vi "Find-NoClasses.vi"() -> ()   [LabVIEW 2016]
uses:
  D:/Users/blume/Desktop/LV/MongoDB-Driver/MLV DLLs/MongoLabVIEW.dll
  LV/MongoDB-Driver/MLV DLLs/MongoLabVIEW.dll
  HITRAN-Line-Cluster.ctl
panel:
  out "Lines":T1[](array[typedef]) {"trans_nu" format="%#.6g"}
  out "Find":string[](array[string])
  out "# lines":i32
  out "convertionTime (ms)":u32
  out "selectionTime (ms)":u32
  in  "selectionString":string="{ _id: false }"
  in  "filterString":string="{ trans_nu: { $gte: 7246, $lte: 7352 }, trans_molec_id: 1 }"
  in  "sortString":string="{param_intensity_weighted_abundace: -1}"
  in  "limitInteger":i32=100
  out "GetNumberOfDocs":i64
  in  "collectionName":string="hitran_2012"
  in  "databaseName":string="hitran"
  in  "connectionString":string="mongodb://tulpe:27017"
  # "MongoDB Example"
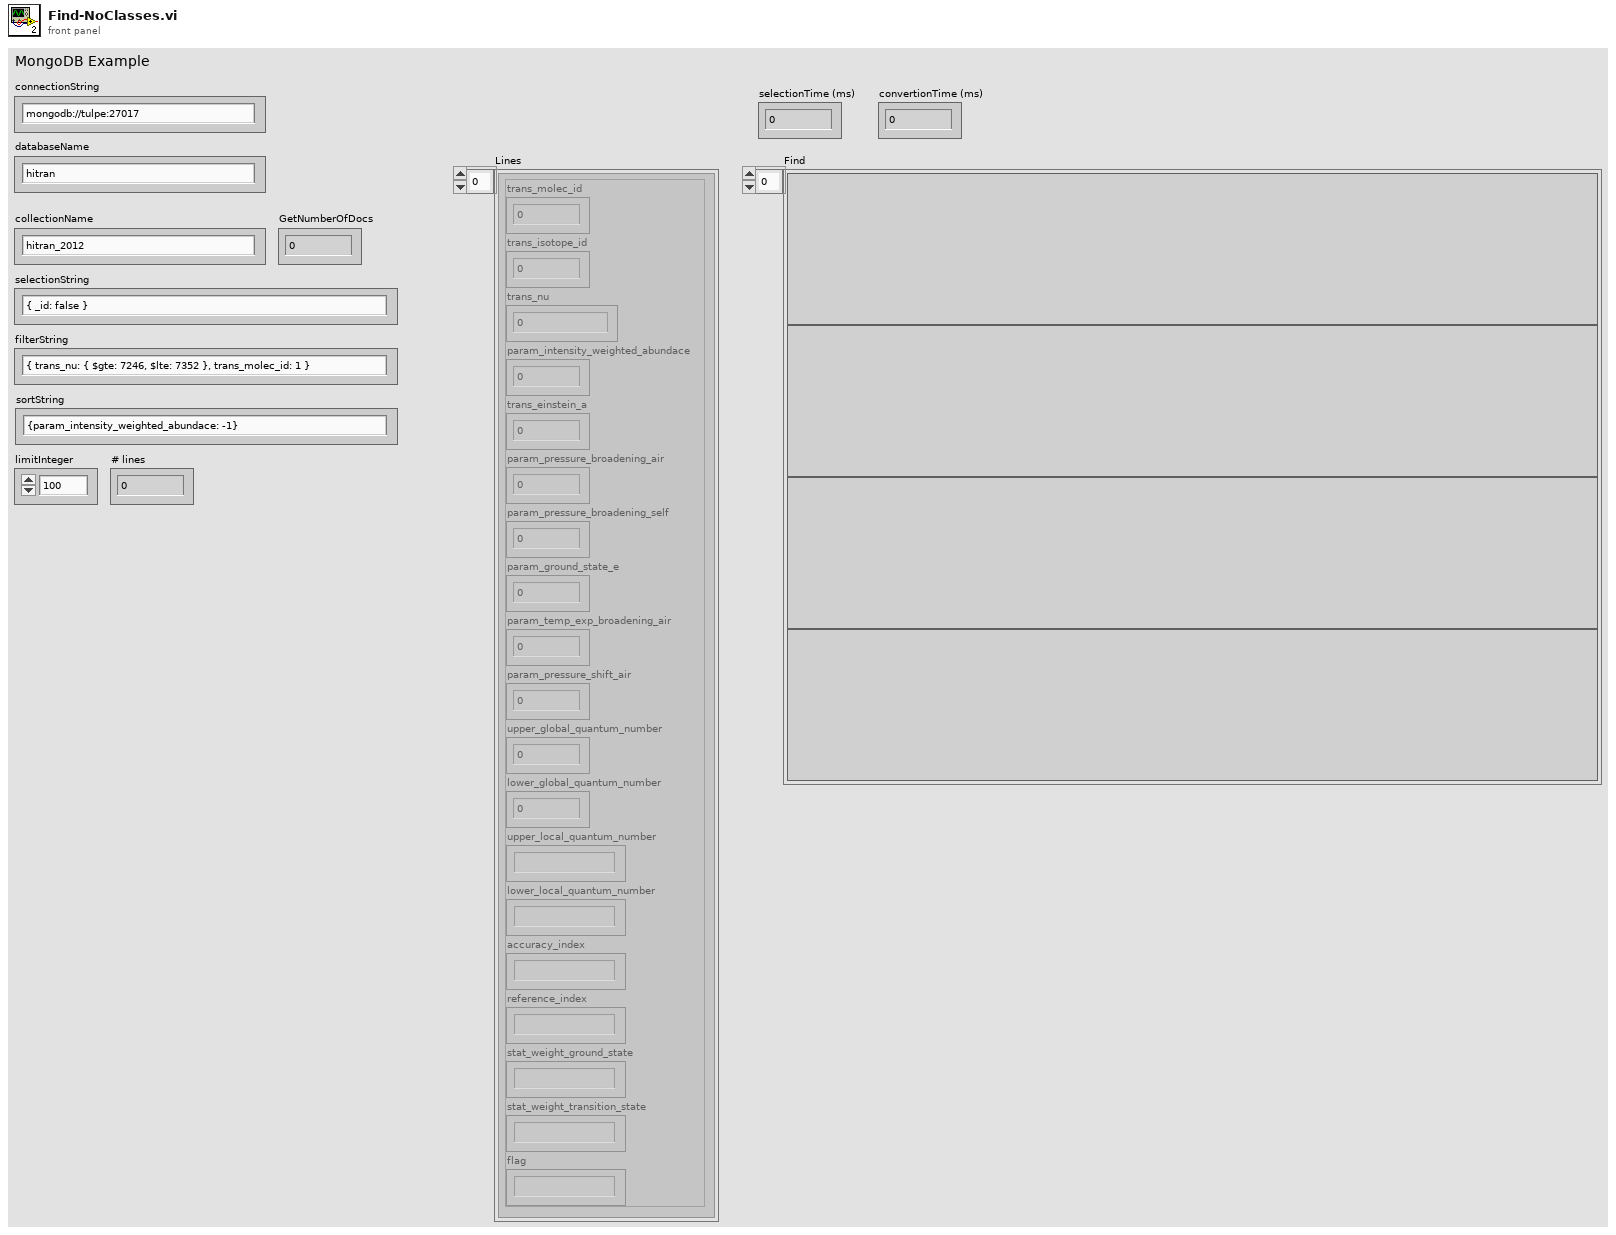
[diagram p1: front panel]
types:
  T1 = typedef "HITRAN-Line-Cluster.ctl" = cluster{"trans_molec_id":i32, "trans_isotope_id":i32, "trans_nu":dbl, "param_intensity_weighted_abundace":dbl, "trans_einstein_a":dbl, "param_pressure_broadening_air":dbl, "param_pressure_broadening_self":dbl, "param_ground_state_e":dbl, "param_temp_exp_broadening_air":dbl, "param_pressure_shift_air":dbl, "upper_global_quantum_number":i32, "lower_global_quantum_number":i32, "upper_local_quantum_number":string, "lower_local_quantum_number":string, "accuracy_index":string, "reference_index":string, "stat_weight_ground_state":string, "stat_weight_transition_state":string, "flag":string}
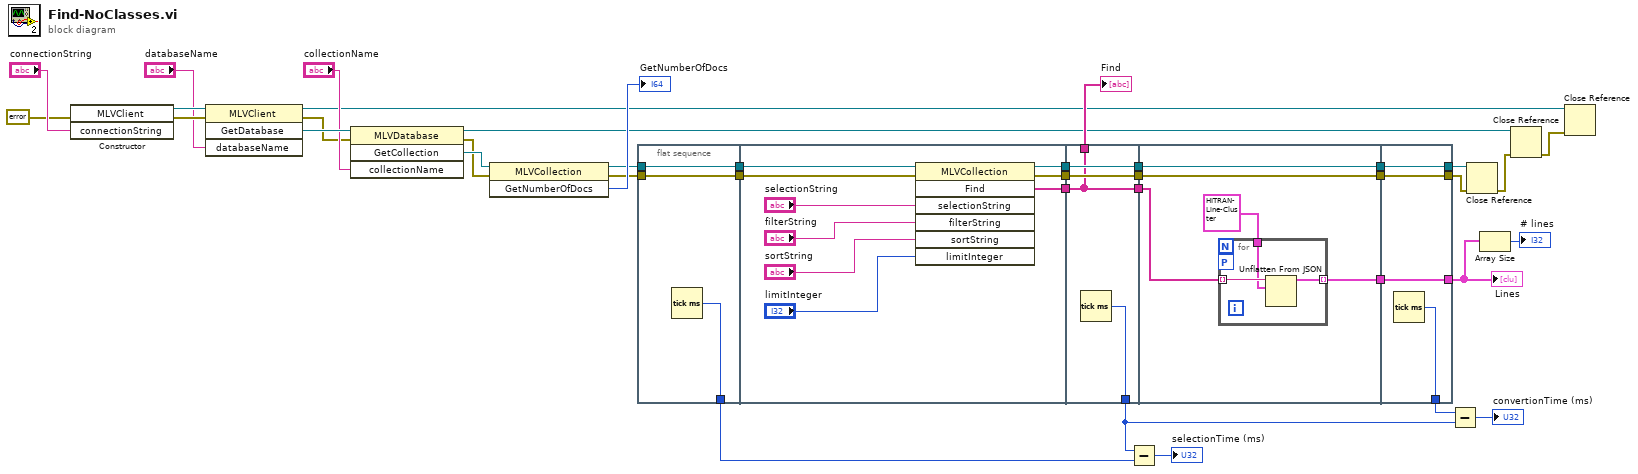
[diagram p0: block diagram]
diagram:
  n1 = constructor class="MLVClient"(error in=errorcluster {"status"=FALSE, "code"=0, "source"=""} ("error in (no error)"), "connectionString"="connectionString") -> (reference out=w18:refnum<k24>, error out=w17:errorcluster)  [unwired: 2 in, 2 out]
  n2 = invoke class="MLVClient" method="GetDatabase"(reference=w18, error in=w17, "databaseName"="databaseName") -> (reference out=w2:refnum<k24>, error out=w13:errorcluster, "GetDatabase"=w15:refnum<k24>)  [unwired: 1 in, 1 out]
  n3 = invoke class="MLVDatabase" method="GetCollection"(reference=w15, error in=w13, "collectionName"="collectionName") -> (reference out=w5:refnum<k24>, error out=w11:errorcluster, "GetCollection"=w12:refnum<k24>)  [unwired: 1 in, 1 out]
  n4 = invoke class="MLVCollection" method="GetNumberOfDocs"(reference=w12, error in=w11) -> (reference out=w8:refnum<k24>, error out=w6:errorcluster, "GetNumberOfDocs"=→"GetNumberOfDocs":i64)  [unwired: 1 in]
  n5 = flat-sequence {
    tunnel: [w41] -> w27
    tunnel: [w40] -> w9
    tunnel: w8 -> [w40]
    tunnel: w6 -> [w39]
    tunnel: [w39] -> w7
    tunnel: [w44] -> w38
    tunnel: [w43] -> w37
    tunnel: [w42] -> w36
    tunnel: w9 -> [w50]
    tunnel: w7 -> [w49]
    tunnel: w38 -> [w54]
    tunnel: w37 -> [w53]
    tunnel: w36 -> [w51]
    tunnel: [w54] -> w35
    tunnel: [w53] -> w34
    tunnel: [w51] -> w33
    tunnel: [w52] -> w25
    tunnel: [w51] -> w20
    tunnel: w35 -> [w59]
    tunnel: w34 -> [w58]
    tunnel: w33 -> [w57]
    tunnel: [w59] -> w32
    tunnel: [w58] -> w31
    tunnel: [w56] -> w30
    tunnel: [w64] -> w22
    tunnel: [w65] -> w28
    tunnel: [w66] -> w29
    tunnel: w32 -> [w66]
    tunnel: w31 -> [w65]
    tunnel: w30 -> [w64]
    tunnel: [w63] -> w26
    frame #0 {
      n6 = Tick Count (ms)() -> (millisecond timer value=w41:u32)
    }
    frame #1 {
      n7 = invoke class="MLVCollection" method="Find"(reference=w50, error in=w49, "selectionString"="selectionString", "filterString"="filterString", "sortString"="sortString", "limitInteger"="limitInteger") -> (reference out=w44:refnum<k24>, error out=w43:errorcluster, "Find"=w42:string[])  [unwired: 1 in, 4 out]
    }
    frame #2 {
      n8 = Tick Count (ms)() -> (millisecond timer value=w52:u32)
    }
    frame #3 {
      n9 = for {
        tunnel: T1 {"trans_molec_id"=0, "trans_isotope_id"=0, "trans_nu"=0.0, "param_intensity_weighted_abundace"=0.0, "trans_einstein_a"=0.0, "param_pressure_broadening_air"=0.0, "param_pressure_broadening_self"=0.0, "param_ground_state_e"=0.0, "param_temp_exp_broadening_air"=0.0, "param_pressure_shift_air"=0.0, "upper_global_quantum_number"=0, "lower_global_quantum_number"=0, "upper_local_quantum_number"="", "lower_local_quantum_number"="", "accuracy_index"="", "reference_index"="", "stat_weight_ground_state"="", "stat_weight_transition_state"="", "flag"=""} ("HITRAN-Line-Cluster") -> [w60]
        tunnel: [w62] -> w56 mode=indexing
        tunnel: w57 -> [w61] mode=indexing
        workers-P: _ -> [_]
        n10 = Unflatten From JSON(JSON string=w61, type and defaults=w60) -> (value=w62:T1)  [unwired: 5 in, 1 out]
      }
    }
    frame #4 {
      n11 = Tick Count (ms)() -> (millisecond timer value=w63:u32)
    }
  }
  n12 = Subtract(x=w25, y=w27) -> (x-y=→"selectionTime (ms)":u32)
  n13 = Subtract(x=w26, y=w25) -> (x-y=→"convertionTime (ms)":u32)
  n14 = Close Reference(reference=w29, error in (no error)=w28) -> (error out=w4:errorcluster)
  n15 = Array Size(array=w22) -> (size(s)=→"# lines":i32)
  n16 = Close Reference(reference=w5, error in (no error)=w4) -> (error out=w3:errorcluster)
  n17 = Close Reference(reference=w2, error in (no error)=w3) -> ()  [unwired: 1 out]
  "Find" <- w20
  "Lines" <- w22
